vi "OKNG IO.vi"(8 "error in (no error)":errorcluster, 11 "Data In":T1) -> (0 "error out":errorcluster, 3 "Data Out":T1)   [LabVIEW 2013]
uses:
  controls/Data.ctl
panel:
  # "日期"
  # "機種名稱"
  # "機種代號"
  # "商品條碼"
  # "OK"
  # "台"
  # "NG"
  # "總計"
  # "台"
  # "日期"
  # "機種名稱"
  # "機種代號"
  # "商品條碼"
  # "OK"
  # "台"
  # "NG"
  # "總計"
  # "台"
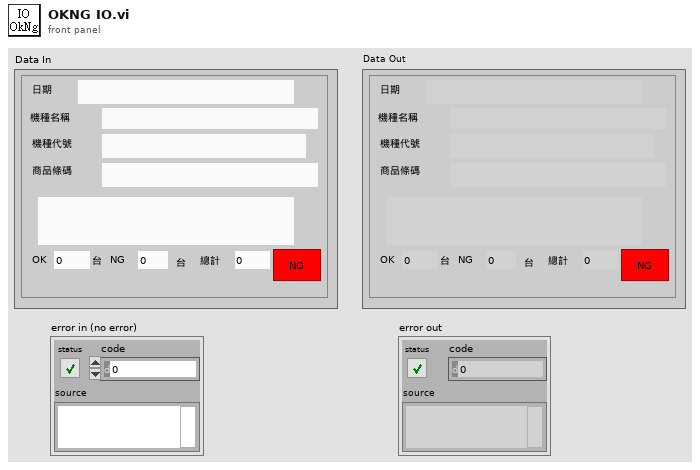
[diagram p1: front panel]
types:
  T1 = typedef "Data.ctl" = cluster{"Date":string, "BarCode1":string, "BarCode2":string, "BarCode3":string, "Message":string, "OK Count":u16, "NG Count":u16, "Total Count":u16, "ModelData":string[][], "OK&NG":bool, "COM1":refnum<visa-resource-name>, "COM2":refnum<visa-resource-name>, "IO":i32, "Time":u32, "TCP":refnum<k5>}
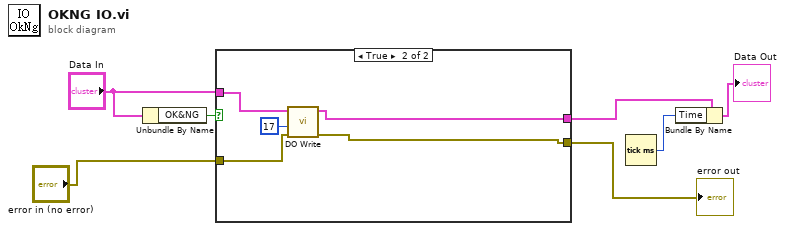
[diagram p0: block diagram]
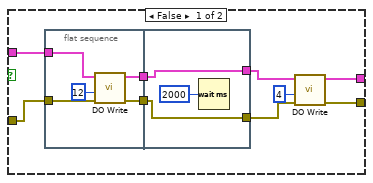
[diagram p2: hidden frame]
diagram:
  n1 = Unbundle By Name("Data In") -> ("OK&NG"=w7:bool)
  n2 = case shown="True" w7 {
    tunnel: "Data In" -> [w16 w29]
    tunnel: "error in (no error)" -> [w15 w27]
    tunnel: [w11 w26] -> w3
    tunnel: [w9 w25] -> w4
    frame False {
      n3 = flat-sequence {
        tunnel: w16 -> [w21]
        tunnel: w15 -> [w20]
        tunnel: [w18] -> w14
        tunnel: [w17] -> w13
        tunnel: w14 -> [w23]
        tunnel: w13 -> [w22]
        tunnel: [w23] -> w12
        tunnel: [w22] -> w10
        frame #0 {
          n4 = call "DO Write.vi"("error in (no error)"=w20, "data"=u8 12, "Data In"=w21) -> ("error out"=w17:errorcluster, "Data Out"=w18:T1)  [unwired: 7 in]
        }
        frame #1 {
          n5 = Wait (ms)(milliseconds to wait=u32 2000) -> ()  [unwired: 1 out]
        }
      }
      n6 = call "DO Write.vi"("error in (no error)"=w10, "data"=u8 4, "Data In"=w12) -> ("error out"=w9:errorcluster, "Data Out"=w11:T1)  [unwired: 7 in]
    }
    frame True {
      n7 = call "DO Write.vi"("error in (no error)"=w27, "data"=u8 17, "Data In"=w29) -> ("error out"=w25:errorcluster, "Data Out"=w26:T1)  [unwired: 7 in]
    }
  }
  "error out" <- w4
  n8 = Tick Count (ms)() -> (millisecond timer value=w1:u32)
  n9 = Bundle By Name(cluster=w3, "Time"=w1) -> (→"Data Out":T1)
